vi "zurichinstMonitor.vi"(0 "Lock-in Reference":u16(ring) items=["Lock-in 1", "Lock-in 2", "Lock-in 3"]) -> ()   [LabVIEW 2019]
uses:
  Utility/Monitor Communication/zurich_lock_in/zurichinstMonitor.ctl
  Instrument_Setup.vi
  Global/Global Variables/Data_Display_global.vi
  Equipment/Zurich Instruments LabOne/Public/Data/ziGetEventDemodSample.vi
  Equipment/Zurich Instruments LabOne/Zurich Instruments LabOne.lvlib
panel:
  out "Zurich-Lock-In Monitor":T1
  out "X":dbl[](graph)
  out "Y":dbl[](graph)
  out "Theta":dbl[](graph)
  out "R":dbl[](graph)
  in  "Path":path
  out "Adress (out)":string
  out "error out":errorcluster
  in  "error in (no error)":errorcluster
  in  "stop":bool
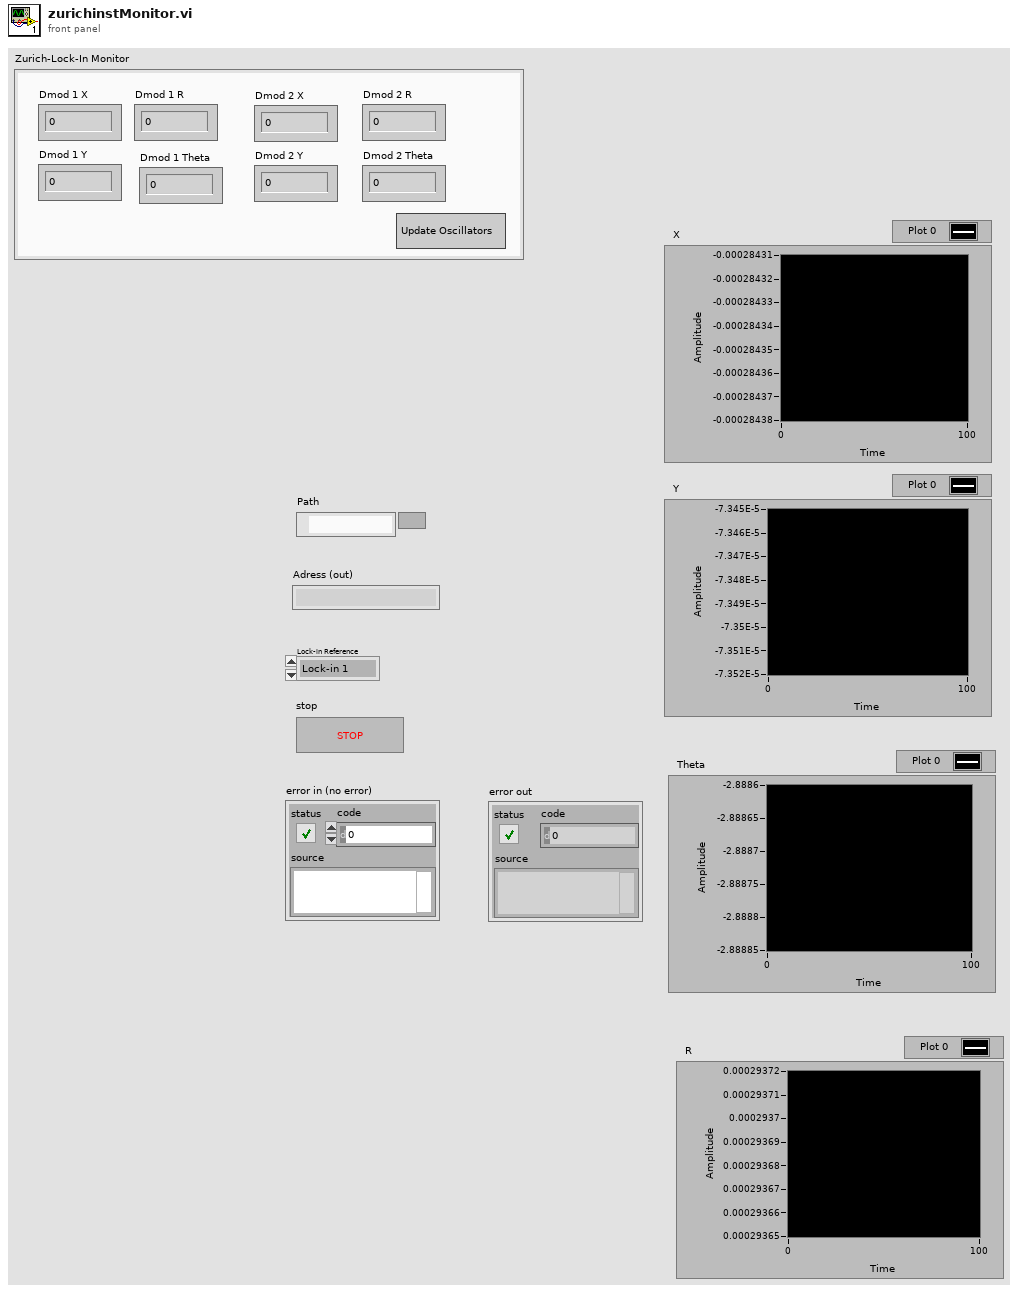
[diagram p1: front panel]
types:
  T1 = typedef "zurichinstMonitor.ctl" = cluster{"Dmod 1 X":dbl, "Dmod 1 Y":dbl, "Dmod 1 R":dbl, "Dmod 1 Theta":dbl, "Update Oscillators":bool, "Dmod 2 X":dbl, "Dmod 2 R":dbl, "Dmod 2 Y":dbl, "Dmod 2 Theta":dbl}
  T2 = typedef "Control 3.ctl" = cluster{"Adress":string, "Load Settings from File":bool, "Output_Demod1":enum16{"Aux 1", "Aux 2", "Aux 3", "Aux 4"}, "Input_Demod1":enum16{"Sig In 1", "Curr In 1", "Trigger 1", "Trigger 2", "Aux Out 1", "Aux Out 2", "Aux Out 3", "Aux Out 4", "Aux In 1", "Aux In 2", "Constant"}, "Input_Mode_Demod1":enum16{"single ended", "differential"}, "Bandwith_Mode_Demod1":enum16{"TC", "BW NEP", "BW 3dB"}, "Bandw_Value_demod1":dbl, "Demod1_Range":dbl, "Demod1_Harmonic":dbl, "Trigger_Demod1":enum16{"Manual", "External"}, "osc1_freq":dbl, "osc1_amp":dbl, "Demod1_scaling":dbl, "osc2_freq":dbl, "osc2_amp":dbl, "osc3_freq":dbl, "osc3_amp":dbl, "osc4_freq":dbl, "osc4_amp":dbl, "Demod1_Phase (deg)":dbl, "Demod1_order":ext, "Demod1_coupling":enum16{"DC", "AC"}, "Demod1_shields":enum16{"Ground", "Float"}, "Demod1_input_resistance":enum16{"10M", "50"}, "Demod1_Ref_oscillator":ext, "Demod1_output_imp":enum16{"Disable", "Enable"}, "Demod1_output_diff":enum16{"Disable", "Enable"}, "Demod1_rate":dbl, "Demod1_Output_range":dbl, "Output_Demod2":enum16{"Aux 1", "Aux 2", "Aux 3", "Aux 4"}, "Demod2_input":enum16{"Sig In 1", "Curr In 1", "Trigger 1", "Trigger 2", "Aux Out 1", "Aux Out 2", "Aux Out 3", "Aux Out 4", "Aux In 1", "Aux In 2", "Constant"}, "Input_Mode_Demod2":enum16{"single ended", "differential"}, "Bandwith_Mode_Demod2":enum16{"TC", "BW NEP", "BW 3dB"}, "Bandw_Value_demod2":dbl, "Demod2_Range":dbl, "Demod2_Harmonic":dbl, "Trigger_Demod2":enum16{"Manual", "External"}, "Demod2_scaling":dbl, "Demod2_Phase (deg)":dbl, "Demod2_order":ext, "Demod2_coupling":enum16{"DC", "AC"}, "Demod2_shields":enum16{"Ground", "Float"}, "Demod2_input_resistance":enum16{"10M", "50"}, "Demod2_Ref_oscillator":ext, "Demod2_output_imp":enum16{"Disable", "Enable"}, "Demod2_output_diff":enum16{"Disable", "Enable"}, "Demod2_rate":dbl, "Demod2_Output_range":dbl, "Output_Demod3":enum16{"Aux 1", "Aux 2", "Aux 3", "Aux 4"}, "Demod3_input":enum16{"Sig In 1", "Curr In 1", "Trigger 1", "Trigger 2", "Aux Out 1", "Aux Out 2", "Aux Out 3", "Aux Out 4", "Aux In 1", "Aux In 2", "Constant"}, "Input_Mode_Demod3":enum16{"single ended", "differential"}, "Bandwith_Mode_Demod2":enum16{"TC", "BW NEP", "BW 3dB"}, "Bandw_Value_demod3":dbl, "Demod3_Range":dbl, "Demod3_Harmonic":dbl, "Trigger_Demod3":enum16{"Manual", "External"}, "Demod3_scaling":dbl, "Demod3_Phase (deg)":dbl, "Demod3_order":ext, "Demod3_coupling":enum16{"DC", "AC"}, "Demod3_shields":enum16{"Ground", "Float"}, "Demod3_input_resistance":enum16{"10M", "50"}, "Demod3_Ref_oscillator":ext, "Demod3_output_imp":enum16{"Disable", "Enable"}, "Demod3_output_diff":enum16{"Disable", "Enable"}, "Demod3_rate":dbl, "Demod3_Output_range":dbl, "Output_Demod4":enum16{"Aux 1", "Aux 2", "Aux 3", "Aux 4"}, "Demod4_input":enum16{"Sig In 1", "Curr In 1", "Trigger 1", "Trigger 2", "Aux Out 1", "Aux Out 2", "Aux Out 3", "Aux Out 4", "Aux In 1", "Aux In 2", "Constant"}, "Input_Mode_Demod4":enum16{"single ended", "differential"}, "Bandwith_Mode_Demod4":enum16{"TC", "BW NEP", "BW 3dB"}, "Bandw_Value_demod4":dbl, "Demod4_Range":dbl, "Demod4_Harmonic":dbl, "Trigger_Demod4":enum16{"Manual", "External"}, "Demod4_scaling":dbl, "Demod4_Phase (deg)":dbl, "Demod4_order":ext, "Demod4_coupling":enum16{"DC", "AC"}, "Demod4_shields":enum16{"Ground", "Float"}, "Demod4_input_resistance":enum16{"10M", "50"}, "Demod4_Ref_oscillator":ext, "Demod4_output_imp":enum16{"Disable", "Enable"}, "Demod4_output_diff":enum16{"Disable", "Enable"}, "Demod4_rate":dbl, "Demod4_Output_range":dbl, "Oscillator1_Amp_units":enum16{"Vpk", "Vrms", "VdBm"}, "Oscillator4_Amp_units":enum16{"Vpk", "Vrms", "VdBm"}, "Oscillator2_Amp_units":enum16{"Vpk", "Vrms", "VdBm"}, "Oscillator3_Amp_units":enum16{"Vpk", "Vrms", "VdBm"}, "Demod1_sync_filter":enum16{"Disable", "Enable"}, "Demod 1 (on/off)":bool, "Demod 2 (on/off) ":bool, "Demod 3 (on/off) ":bool, "Demod 4 (on/off) ":bool, " Sigouts 1 (on/off)":bool, " Sigouts 2 (on/off) ":bool, " Sigouts 3 (on/off)":bool, " Sigouts 4 (on/off) ":bool, "Demod2_sync_filter":enum16{"Disable", "Enable"}, "Demod1_auto_outp_rang":enum16{"Disable", "Enable"}, "Demod2_auto_outp_rang ":enum16{"Disable", "Enable"}}
  T3 = typedef "Zurich Instruments LabOne.lvlib/ziTypeHandle.ctl" = cluster{"handleValid":bool, "Conn":u64, "Path Prefix":string, "Handle":u64, "Connected":bool, "Clockbase(s)":dbl}
  T4 = typedef "Zurich Instruments LabOne.lvlib/ziTypePollType.ctl" = enum16{"NONE", "DOUBLE_DATA", "INTEGER_DATA", "DEMOD_SAMPLE", "SCOPE_WAVE_HF2", "AUXIN_SAMPLE", "DIO_SAMPLE", "BYTE_ARRAY", "PWA_WAVE", "9", "10", "11", "12", "13", "14", "15", "TREE_CHANGE_DEPRI", "17", "ERROR", "19", "20", "21", "22", "23", "24", "25", "26", "27", "28", "29", "30", "31", "DOUBLE_DATA_TS", "INTEGER_DATA_TS", "34", "SCOPE_WAVE", "SCOPE_WAVE_EX", "37", "BYTE_ARRAY_TS", "39", "40", "41", "42", "43", "44", "45", "CNT_DATA", "47", "TREE_CHANGE", "49", "50", "51", "52", "53", "54", "55", "56", "57", "58", "59", "60", "61", "62", "63", "SWEEPER_DATA", "SPECTRUM_DATA", "ADVISOR_DATA", "VECTOR_DATA", "IMP_DATA"}
  T5 = typedef "Zurich Instruments LabOne.lvlib/ziTypeDemodSampleEx.ctl" = cluster{"Timestamps (ticks)":u64[], "X (Vrms)":dbl[], "Y (Vrms)":dbl[], "Osc Phase (rad)":dbl[], "Freq (Hz)":dbl[], "DIO":u32[], "Aux In 0 (V)":dbl[], "Aux In 1 (V)":dbl[], "Trigger":u32[]}
  T6 = cluster{"LIA7230-Running":bool, "LIA7230-Running 2":bool, "LIA7230-Running 3":bool, "SR830-Running":bool, "SR830-Running 2":bool, "SR830-Running 3":bool, "PE7265-running":bool, "zurich_Lock_in-running":bool}
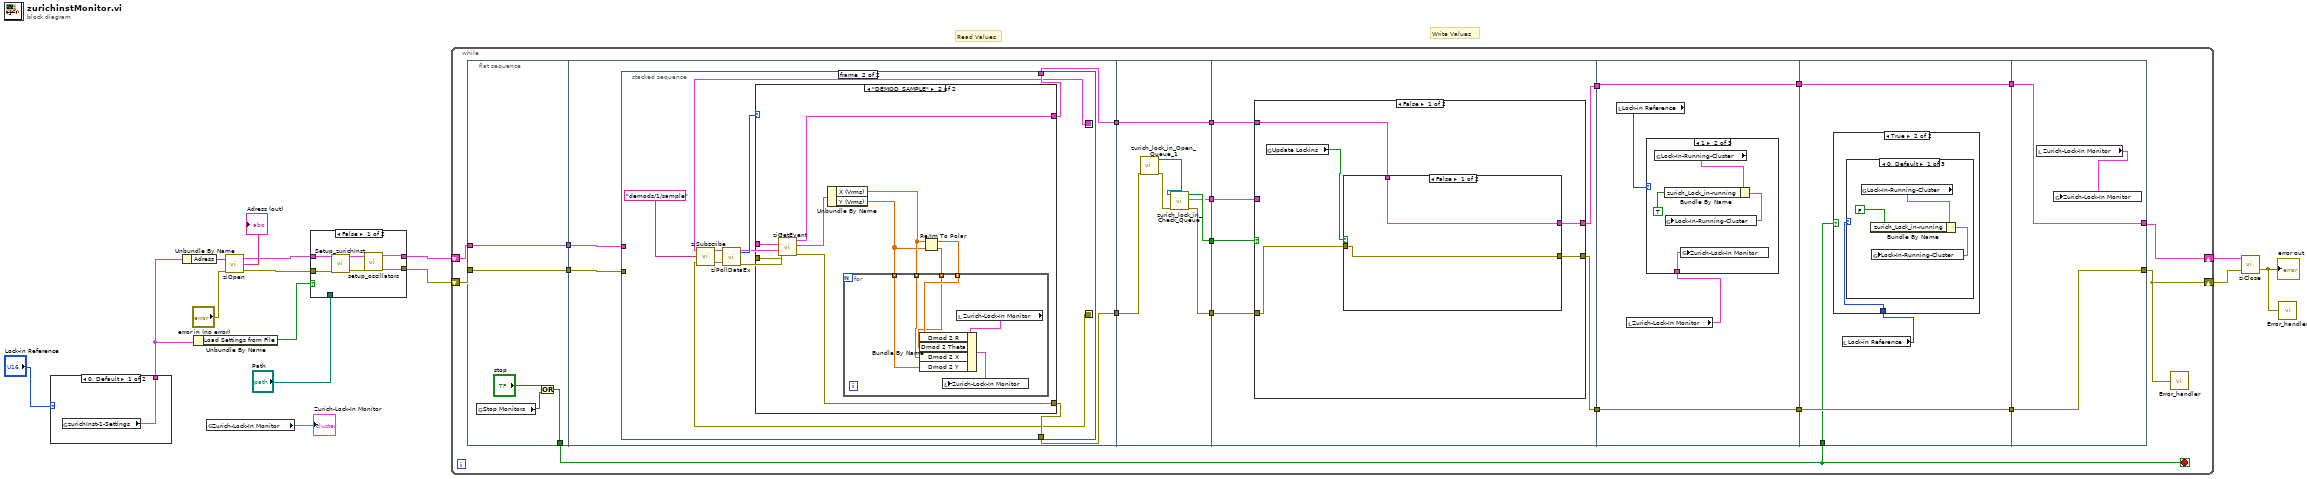
[diagram p0: block diagram]
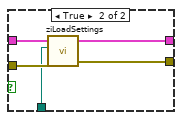
[diagram p2: hidden frame]
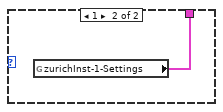
[diagram p3: hidden frame]
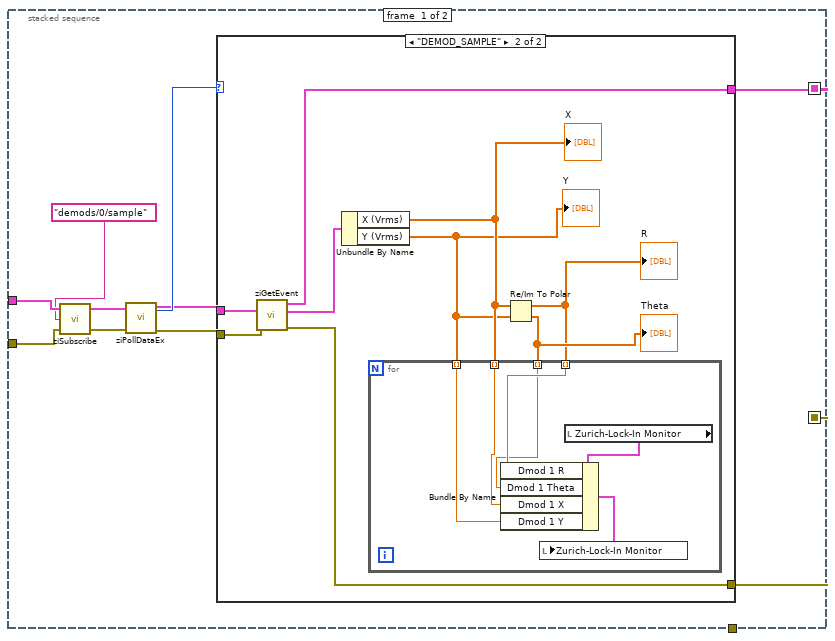
[diagram p4: hidden frame]
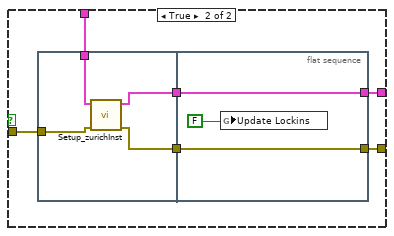
[diagram p7: hidden frame]
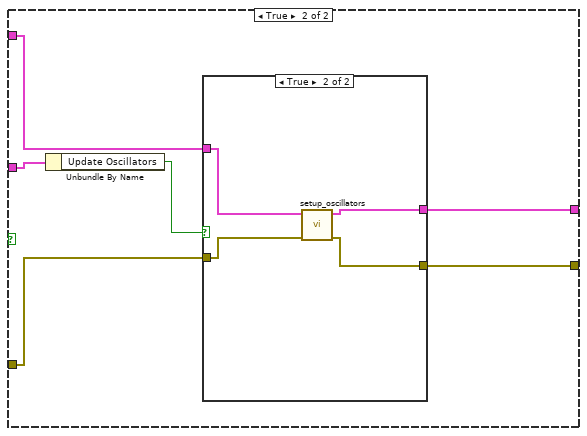
[diagram p8: hidden frame]
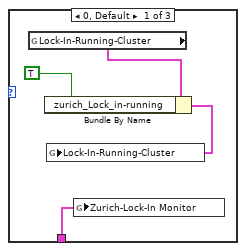
[diagram p10: hidden frame]
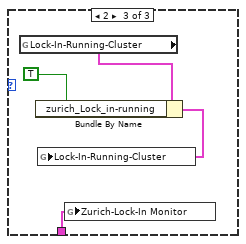
[diagram p11: hidden frame]
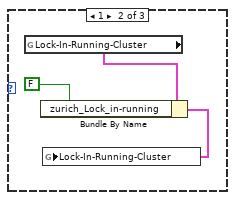
[diagram p13: hidden frame]
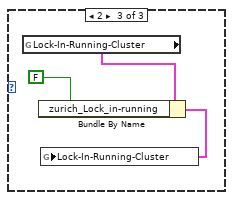
[diagram p14: hidden frame]
diagram:
  # "Write Values"
  # "Read Values"
  n1 = case shown="0, Default" "Lock-in Reference" {
    tunnel: [w16 w17] -> w11
    frame 0, Default {
      n2 = global read "Instrument_Setup.vi" "zurichInst-1-Settings"() -> (w16:T2)
    }
    frame 1 {
      n3 = global read "Instrument_Setup.vi" "zurichInst-1-Settings"() -> (w17:T2)
    }
  }
  n4 = Unbundle By Name(w11) -> ("Adress"=w14:string)
  n5 = Unbundle By Name(w11) -> ("Load Settings from File"=w10:bool)
  n6 = global read "Data_Display_global.vi" "Zurich-Lock-In Monitor"() -> (→"Zurich-Lock-In Monitor":T1)
  n7 = call "ziOpen.vi"("Error In"="error in (no error)", "Address"=w14) -> ("Error Out"=w3:errorcluster, "Selected Device"=→"Adress (out)":string, "HandleOut"=w4:T3)  [unwired: 2 in]
  n8 = case shown="False" w10 {
    tunnel: w4 -> [w23 w28]
    tunnel: [w19 w27] -> w2
    tunnel: w3 -> [w22 w26]
    tunnel: [w18 w25] -> w1
    tunnel: "Path" -> [_ w24]
    frame False {
      n9 = call "Setup_zurichInst.vi"("error in (no error)"=w22, "Handle In"=w23) -> ("error out"=w20:errorcluster, "Handle Out"=w21:T3)  [unwired: 8 in]
      n10 = call "setup_oscillators.vi"("error in (no error)"=w20, "Handle In"=w21) -> ("error out"=w18:errorcluster, "Handle Out"=w19:T3)  [unwired: 8 in]
    }
    frame True {
      n11 = call "ziLoadSettings.vi"("Error in"=w26, "File path (dialog if empty)"=w24, "Handle in"=w28) -> ("Error out"=w25:errorcluster, "Handle out"=w27:T3)  [unwired: 2 in]
    }
  }
  n12 = while {
    shift-right: [w47] -> w8
    shift-left: w1 -> [w45]
    shift-right: [w36] -> w6
    shift-left: w2 -> [w43]
    stop <- w29 stop-if-true
    n13 = flat-sequence {
      tunnel: [w50] -> w29
      tunnel: [w49] -> w46
      tunnel: w45 -> [w49]
      tunnel: [w48] -> w44
      tunnel: w43 -> [w48]
      tunnel: w46 -> [w53]
      tunnel: w44 -> [w54]
      tunnel: [w56] -> w41
      tunnel: [w55] -> w39
      tunnel: [w117] -> w42
      tunnel: w41 -> [w117]
      tunnel: [w112] -> w40
      tunnel: w39 -> [w116]
      tunnel: [w114] -> w38
      tunnel: [w111] -> w37
      tunnel: w42 -> [w123]
      tunnel: w40 -> [w122]
      tunnel: w38 -> [w121]
      tunnel: w37 -> [w120]
      tunnel: [w119] -> w35
      tunnel: [w118] -> w34
      tunnel: w35 -> [w159]
      tunnel: [w159] -> w33
      tunnel: w34 -> [w158]
      tunnel: [w158] -> w31
      tunnel: w33 -> [w175]
      tunnel: [w175] -> w32
      tunnel: w31 -> [w174]
      tunnel: [w174] -> w30
      tunnel: w29 -> [w173]
      tunnel: [w187] -> w47
      tunnel: [w188] -> w36
      tunnel: w32 -> [w188]
      tunnel: w30 -> [w187]
      frame #0 {
        n14 = global read "Data_Display_global.vi" "Stop Monitors"() -> (w52:bool)
        n15 = Or(x="stop", y=w52) -> (x .or. y?=w50:bool)
      }
      frame #1 {
        n16 = stacked-sequence {
          seq-local: [w63 _] -> [_ w84]
          seq-local: [w62 _] -> [_ w85]
          tunnel: w54 -> [w59 _]
          tunnel: w53 -> [w58 _]
          tunnel: [_ w87] -> w56
          tunnel: [_ w86] -> w55
          frame #0 {
            n17 = call "ziSubscribe.vi"("error in"=w58, "Path ()"="demods/0/sample", "Handle In"=w59) -> ("error out"=w60:errorcluster, "Handle Out"=w61:T3)  [unwired: 1 in]
            n18 = call "ziPollDataEx.vi"("error in"=w60, "Handle In"=w61) -> ("error out"=w64:errorcluster, "Handle Out"=w65:T3, "ziValueType"=w66:T4)  [unwired: 2 in, 5 out]
            n19 = case shown="\"DEMOD_SAMPLE\"" w66 {
              tunnel: w65 -> [w68 w77]
              tunnel: w64 -> [w67 w76]
              tunnel: [w68 w70] -> w63
              tunnel: [w67 w69] -> w62
              frame "NONE", Default {
              }
              frame "DEMOD_SAMPLE" {
                n20 = call-poly "ziGetEvent.vi"("Error In"=w76, "Handle In"=w77) -> ("Error Out"=w69:errorcluster, "Demod Sample Out"=w75:T5, "Handle Out"=w70:T3)  [unwired: 7 in]
                n21 = Unbundle By Name(w75) -> ("X (Vrms)"=w74:dbl[], "Y (Vrms)"=w73:dbl[])
                "X" <- w74
                "Y" <- w73
                n22 = Re/Im To Polar(2:w73, 3:w74) -> (0:w72:dbl[], 1:w71:dbl[])
                "Theta" <- w72
                "R" <- w71
                n23 = for {
                  tunnel: w73 -> [w78] mode=indexing
                  tunnel: w74 -> [w79] mode=indexing
                  tunnel: w72 -> [w80] mode=indexing
                  tunnel: w71 -> [w81] mode=indexing
                  n24 = local read "Zurich-Lock-In Monitor"() -> (w83:T1)
                  n25 = Bundle By Name(cluster=w83, "Dmod 1 R"=w81, "Dmod 1 Theta"=w80, "Dmod 1 X"=w79, "Dmod 1 Y"=w78) -> (w82:T1)
                  n26 = local write "Zurich-Lock-In Monitor"(w82) -> ()
                }
              }
            }
          }
          frame #1 {
            n27 = call "ziSubscribe.vi"("error in"=w85, "Path ()"="demods/1/sample", "Handle In"=w84) -> ("error out"=w89:errorcluster, "Handle Out"=w90:T3)  [unwired: 1 in]
            n28 = call "ziPollDataEx.vi"("error in"=w89, "Handle In"=w90) -> ("error out"=w91:errorcluster, "Handle Out"=w92:T3, "ziValueType"=w93:T4)  [unwired: 2 in, 5 out]
            n29 = case shown="\"DEMOD_SAMPLE\"" w93 {
              tunnel: w92 -> [w95 w104]
              tunnel: w91 -> [w94 w103]
              tunnel: [w95 w97] -> w87
              tunnel: [w94 w96] -> w86
              frame "NONE", Default {
              }
              frame "DEMOD_SAMPLE" {
                n30 = call-poly "ziGetEvent.vi"("Error In"=w103, "Handle In"=w104) -> ("Error Out"=w96:errorcluster, "Demod Sample Out"=w102:T5, "Handle Out"=w97:T3)  [unwired: 7 in]
                n31 = Unbundle By Name(w102) -> ("X (Vrms)"=w101:dbl[], "Y (Vrms)"=w100:dbl[])
                n32 = Re/Im To Polar(2:w100, 3:w101) -> (0:w99:dbl[], 1:w98:dbl[])
                n33 = for {
                  tunnel: w100 -> [w105] mode=indexing
                  tunnel: w101 -> [w106] mode=indexing
                  tunnel: w99 -> [w107] mode=indexing
                  tunnel: w98 -> [w108] mode=indexing
                  n34 = local read "Zurich-Lock-In Monitor"() -> (w110:T1)
                  n35 = Bundle By Name(cluster=w110, "Dmod 2 R"=w108, "Dmod 2 Theta"=w107, "Dmod 2 X"=w106, "Dmod 2 Y"=w105) -> (w109:T1)
                  n36 = local write "Zurich-Lock-In Monitor"(w109) -> ()
                }
              }
            }
          }
        }
      }
      frame #2 {
        n37 = call "zurich_lock_in_Open_Queue_1.vi"("error in (no error)"=w116) -> ("error out"=w113:errorcluster, "queue out"=w115:refnum<queue>)  [unwired: 9 in]
        n38 = call "zurich_lock_in_Check_Queue.vi"("error in (no error)"=w113, "queue"=w115) -> ("error out"=w112:errorcluster, "Zurich-Lock-In Monitor"=w111:T1, "New Entries?"=w114:bool)  [unwired: 7 in]
      }
      frame #3 {
        n39 = case shown="False" w121 {
          tunnel: w123 -> [w127 w147]
          tunnel: [w126 w145] -> w119
          tunnel: w122 -> [w125 w146]
          tunnel: [w124 w144] -> w118
          tunnel: w120 -> [_ w149]
          frame False {
            n40 = global read "Instrument_Setup.vi" "Update Lockins"() -> (w128:bool)
            n41 = case shown="False" w128 {
              tunnel: w127 -> [w130 w136]
              tunnel: [w130 w134] -> w126
              tunnel: w125 -> [w129 w133]
              tunnel: [w129 w131] -> w124
              frame False {
              }
              frame True {
                n42 = flat-sequence {
                  tunnel: w136 -> [w140]
                  tunnel: [w139] -> w135
                  tunnel: w133 -> [w138]
                  tunnel: [w137] -> w132
                  tunnel: [w142] -> w134
                  tunnel: w135 -> [w142]
                  tunnel: [w141] -> w131
                  tunnel: w132 -> [w141]
                  frame #0 {
                    n43 = call "Setup_zurichInst.vi"("error in (no error)"=w138, "Handle In"=w140) -> ("error out"=w137:errorcluster, "Handle Out"=w139:T3)  [unwired: 8 in]
                  }
                  frame #1 {
                    n44 = global write "Instrument_Setup.vi" "Update Lockins"(FALSE) -> ()
                  }
                }
              }
            }
          }
          frame True {
            n45 = Unbundle By Name(w149) -> ("Update Oscillators"=w148:bool)
            n46 = case shown="True" w148 {
              tunnel: w147 -> [w151 w155]
              tunnel: w146 -> [w150 w154]
              tunnel: [w151 w153] -> w145
              tunnel: [w150 w152] -> w144
              frame False {
              }
              frame True {
                n47 = call "setup_oscillators.vi"("error in (no error)"=w154, "Handle In"=w155) -> ("error out"=w152:errorcluster, "Handle Out"=w153:T3)  [unwired: 8 in]
              }
            }
          }
        }
      }
      frame #4 {
        n48 = local read "Lock-in Reference"() -> (w156:u16)
        n49 = local read "Zurich-Lock-In Monitor"() -> (w157:T1)
        n50 = case shown="1" w156 {
          tunnel: w157 -> [w160 w164 w171]
          frame 0, Default {
            n51 = global read "Data_Display_global.vi" "Lock-In-Running-Cluster"() -> (w163:T6)
            n52 = Bundle By Name(cluster=w163, "zurich_Lock_in-running"=TRUE) -> (w161:T6)
            n53 = global write "Data_Display_global.vi" "Lock-In-Running-Cluster"(w161) -> ()
            n54 = global write "Data_Display_global.vi" "Zurich-Lock-In Monitor"(w160) -> ()
          }
          frame 1 {
            n55 = global read "Data_Display_global.vi" "Lock-In-Running-Cluster"() -> (w167:T6)
            n56 = Bundle By Name(cluster=w167, "zurich_Lock_in-running"=TRUE) -> (w165:T6)
            n57 = global write "Data_Display_global.vi" "Lock-In-Running-Cluster"(w165) -> ()
            n58 = global write "Data_Display_global.vi" "Zurich-Lock-In Monitor"(w164) -> ()
          }
          frame 2 {
            n59 = global read "Data_Display_global.vi" "Lock-In-Running-Cluster"() -> (w170:T6)
            n60 = Bundle By Name(cluster=w170, "zurich_Lock_in-running"=TRUE) -> (w168:T6)
            n61 = global write "Data_Display_global.vi" "Lock-In-Running-Cluster"(w168) -> ()
            n62 = global write "Data_Display_global.vi" "Zurich-Lock-In Monitor"(w171) -> ()
          }
        }
      }
      frame #5 {
        n63 = local read "Lock-in Reference"() -> (w172:u16)
        n64 = case shown="True" w173 {
          tunnel: w172 -> [_ w176]
          frame False {
          }
          frame True {
            n65 = case shown="0, Default" w176 {
              frame 0, Default {
                n66 = global read "Data_Display_global.vi" "Lock-In-Running-Cluster"() -> (w179:T6)
                n67 = Bundle By Name(cluster=w179, "zurich_Lock_in-running"=FALSE) -> (w177:T6)
                n68 = global write "Data_Display_global.vi" "Lock-In-Running-Cluster"(w177) -> ()
              }
              frame 1 {
                n69 = global read "Data_Display_global.vi" "Lock-In-Running-Cluster"() -> (w182:T6)
                n70 = Bundle By Name(cluster=w182, "zurich_Lock_in-running"=FALSE) -> (w180:T6)
                n71 = global write "Data_Display_global.vi" "Lock-In-Running-Cluster"(w180) -> ()
              }
              frame 2 {
                n72 = global read "Data_Display_global.vi" "Lock-In-Running-Cluster"() -> (w185:T6)
                n73 = Bundle By Name(cluster=w185, "zurich_Lock_in-running"=FALSE) -> (w183:T6)
                n74 = global write "Data_Display_global.vi" "Lock-In-Running-Cluster"(w183) -> ()
              }
            }
          }
        }
      }
      frame #6 {
        n75 = local read "Zurich-Lock-In Monitor"() -> (w186:T1)
        n76 = global write "Data_Display_global.vi" "Zurich-Lock-In Monitor"(w186) -> ()
      }
    }
    n77 = call "Error_handler.vi"("error constant"=w47) -> ()
  }
  n78 = call "ziClose.vi"("Error In"=w8, "Handle In"=w6) -> ("Error Out"=w7:errorcluster)  [unwired: 2 in, 1 out]
  "error out" <- w7
  n79 = call "Error_handler.vi"("error constant"=w7) -> ()
